vi "Stop AsyncSum.vi"(8 "error in (no error)":errorcluster, 10 "Opeation":string, 11 "Skeleton in":refnum<class "Skeleton.lvclass">) -> (0 "error out":errorcluster, 3 "Skeleton out":refnum<class "Skeleton.lvclass">)   [LabVIEW 2016, in "Skeleton.lvlib" / "Skeleton.lvclass"]
uses:
  Skeleton.lvclass
  Skeleton.lvclass/Skeleton.ctl
  Active Thread Configuration.ctl
  DemoSkeleton/DemoSkeleton.lvlib
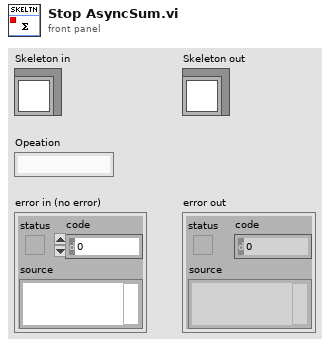
[diagram p1: front panel]
types:
  T1 = typedef "Skeleton.lvlib/Skeleton.lvclass/Active Thread Configuration.ctl" = cluster{"Operation":string, "Handle":u64, "LVUserEvent CallBack Reference":refnum<user-event>}
  T2 = typedef "Skeleton.lvlib/Skeleton.lvclass/Private Data.ctl" = cluster{"DLL path":path, "Active Thread Map":variant}
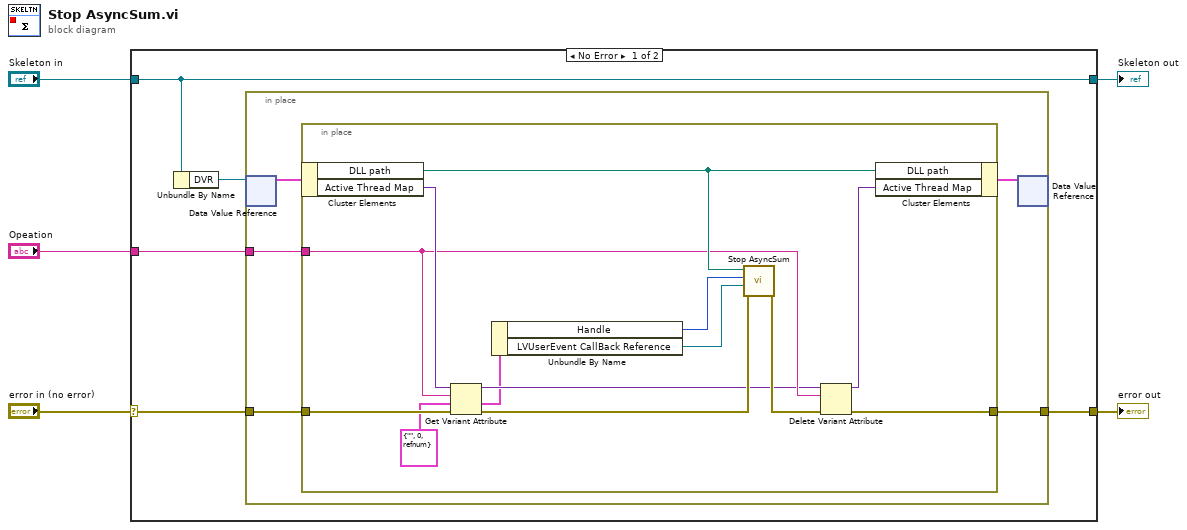
[diagram p0: block diagram]
diagram:
  n1 = case shown="No Error" "error in (no error)" {
    selector: "error in (no error)" -> [w9 w30]
    tunnel: [w8 w30] -> w4
    tunnel: [w10 w29] -> w2
    tunnel: "Skeleton in" -> [w10 w29]
    tunnel: "Opeation" -> [w6 _]
    frame No Error {
      n2 = Unbundle By Name(w10) -> ("DVR"=w7:refnum<data-value>)
      n3 = in-place {
        in-place-border: w9 -> [w15]
        in-place-border: [w14] -> w8
        in-place-border: w6 -> [w11]
        n4 = in-place-dvr #1(w7) -> (w13:T2)  [unwired: 1 out]
        n5 = in-place {
          in-place-border: w15 -> [w25]
          in-place-border: [w21] -> w14
          in-place-border: w11 -> [w26]
          n6 = in-place-cluster #2(w13) -> ("DLL path"=w28:path, "Active Thread Map"=w27:variant)
          n7 = Get Variant Attribute(Variant=w27, name=w26, default value (empty Variant)=T1 {"Operation"="", "Handle"=0, "LVUserEvent CallBack Reference"=refnum} ("Active Thread Configuration"), error in=w25) -> (duplicate Variant=w20:variant, value=w18:T1, error out=w23:errorcluster)  [unwired: 1 out]
          n8 = Unbundle By Name(w18) -> ("Handle"=w17:u64, "LVUserEvent CallBack Reference"=w16:refnum<user-event>)
          n9 = call "Stop AsyncSum.vi"("error in (no error)"=w23, "LVUserEventCallBackRef"=w16, "Handle"=w17, "path in"=w28) -> ("error out"=w22:errorcluster)  [unwired: 6 in, 1 out]
          n10 = Delete Variant Attribute(4:w22, 6:w26, 7:w20) -> (0:w21:errorcluster, 3:w19:variant)  [unwired: 1 out]
          n11 = in-place-cluster #2("DLL path"=w28, "Active Thread Map"=w19) -> (w12:T2)
        }
        n12 = in-place-dvr #1(w12) -> ()  [unwired: 2 out]
      }
    }
    frame Error {
    }
  }
  "error out" <- w4
  "Skeleton out" <- w2
